vi "read37 and record.vi"(3 "Interval_ms":dbl, 4 "VISA资源名称":refnum<visa-resource-name>) -> (1 "本次记录到的字符串":string)   [LabVIEW 2017]
uses:
  <vilib>/Instr/_visa.llb/VISA Configure Serial Port (Instr).vi
  <vilib>/addons/Tools/Unicode/UTF8 Tools.lvlib
panel:
  out "sensor1":dbl[](array[numeric])
  out "SENSOR21":dbl[](array[numeric])
  out "SENSOR25":dbl[](array[numeric])
  out "SENDSOR13":dbl[](array[numeric])
  out "SENSOR15":dbl[](array[numeric])
  out "SENSOR5":dbl[](array[numeric])
  out "SNESOR3":dbl[](array[numeric])
  out "SENSOR23":dbl[](array[numeric])
  out "SENSOR11":dbl[](array[numeric])
  out "错误输出 2":errorcluster caption="错误输出"
  in  "?":enum32{"CONTROL", "选项卡 2"}(tab)
  in  "增益选择":u16(ring) items=["±6.144V", "±4.096V", "±2.048V", "±1.024V", "±0.512V", "±0.256V"]
  in  "连接方式":u16(ring) items=["Serial", "WiFi", "Dual"]
  out "数值显示控件 37":dbl
  out "数值显示控件":dbl
  out "数值显示控件 2":dbl
  out "数值显示控件 3":dbl
  out "SENSOR11":dbl format="%#.2f"
  out "数值显示控件 5":dbl
  out "数值显示控件 6":dbl
  out "SENSOR13":dbl format="%#.2f"
  out "数值显示控件 8":dbl
  out "数值显示控件 9":dbl
  out "数值显示控件 10":dbl
  out "SENSOR25":dbl format="%#.2f"
  out "数值显示控件 12":dbl
  out "数值显示控件 13":dbl
  out "数值显示控件 14":dbl
  out "SENSOR15":dbl format="%#.2f"
  out "SENSOR5":dbl format="%#.2f"
  out "数值显示控件 17":dbl
  out "数值显示控件 18":dbl
  out "SENSOR23":dbl format="%#.2f"
  out "数值显示控件 20":dbl
  out "数值显示控件 21":dbl
  out "数值显示控件 22":dbl
  out "SENSOR21":dbl format="%#.2f"
  out "数值显示控件 24":dbl
  out "SENSOR1":dbl format="%#.2g"
  out "数值显示控件 26":dbl
  out "数值显示控件 27":dbl
  out "数值显示控件 28":dbl
  out "数值显示控件 29":dbl
  out "数值显示控件 30":dbl
  out "SENSOR3":dbl format="%#.2f"
  out "数值显示控件 32":dbl
  out "数值显示控件 33":dbl
  out "数值显示控件 34":dbl
  out "数值显示控件 35":dbl
  out "数值显示控件 36":dbl
  out "本次":string
  out "finally":string[][](array[string])
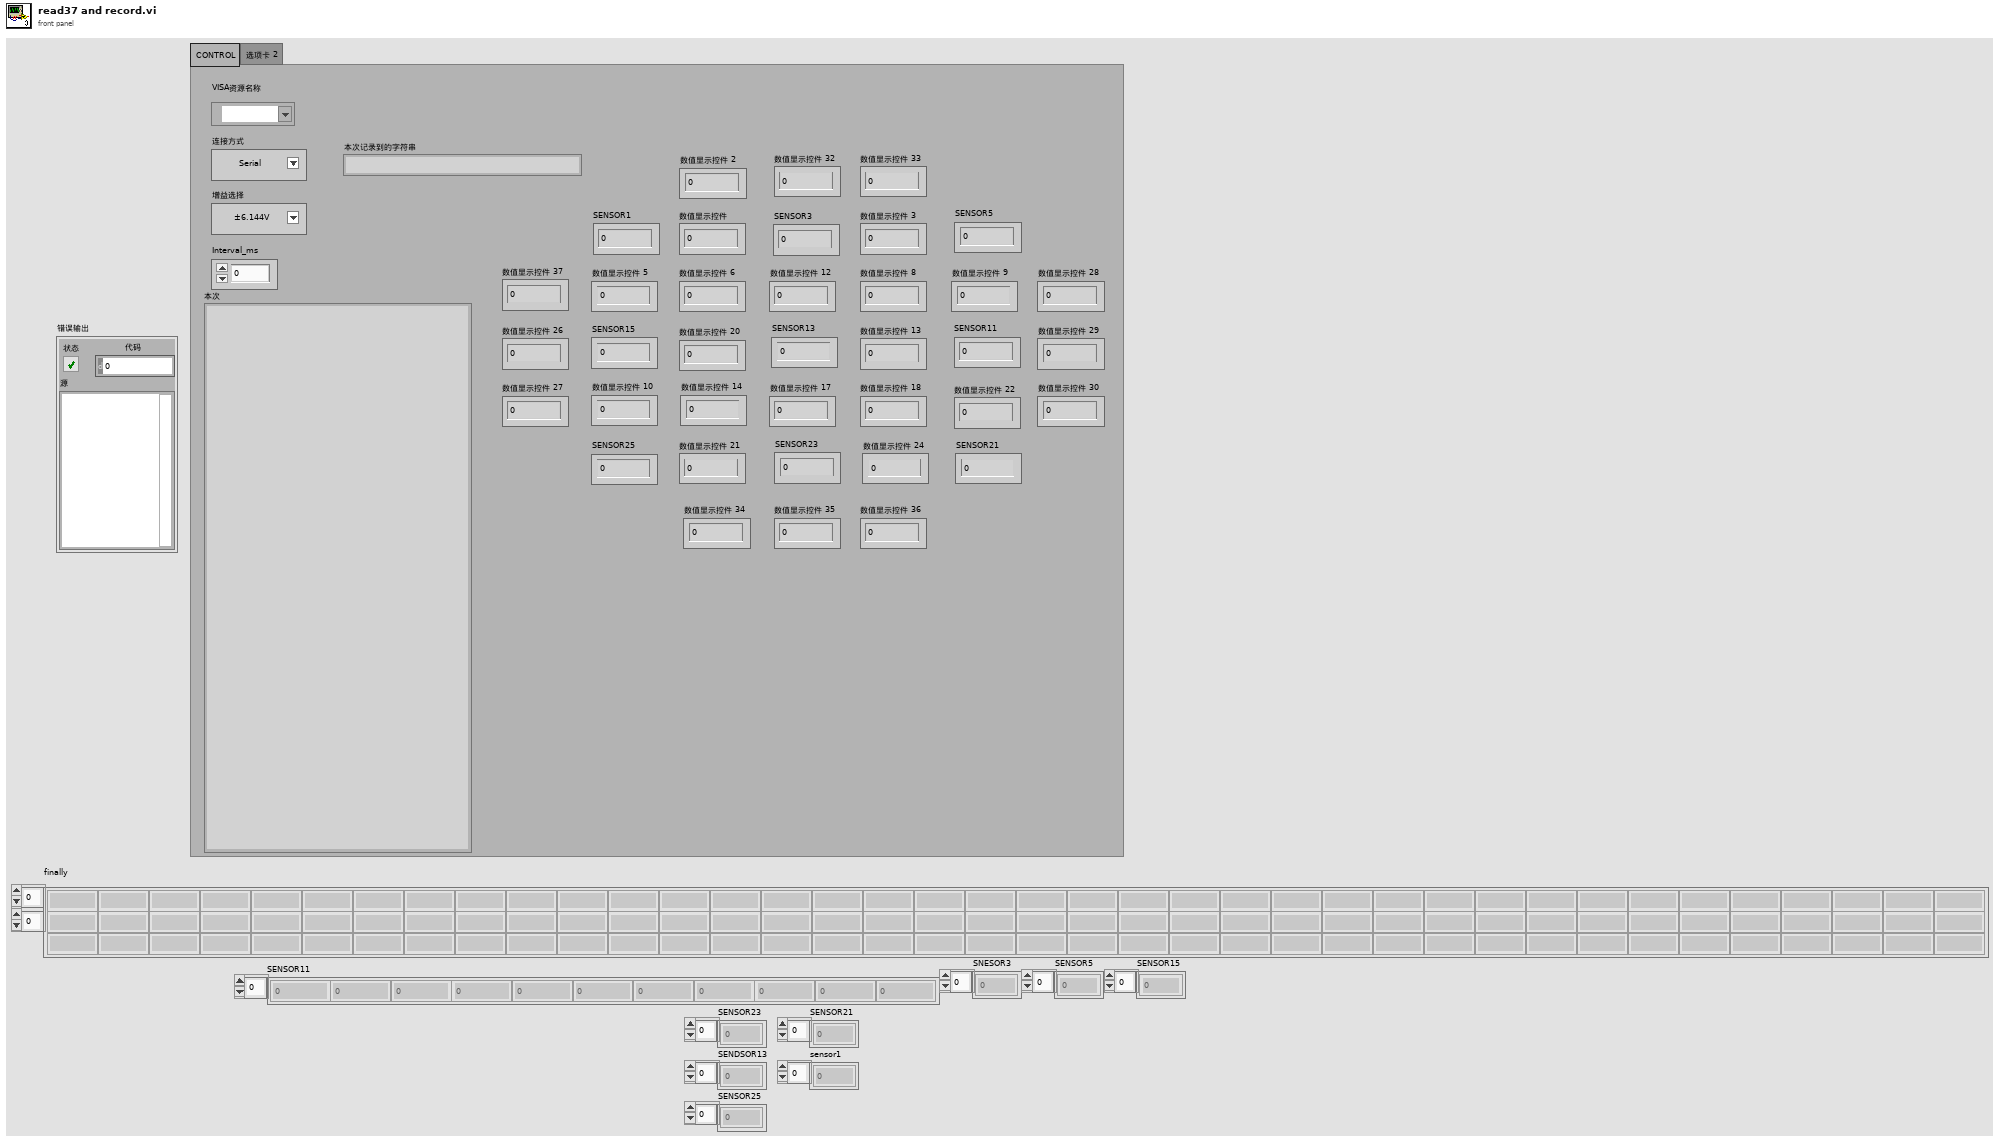
[diagram p1: front panel]
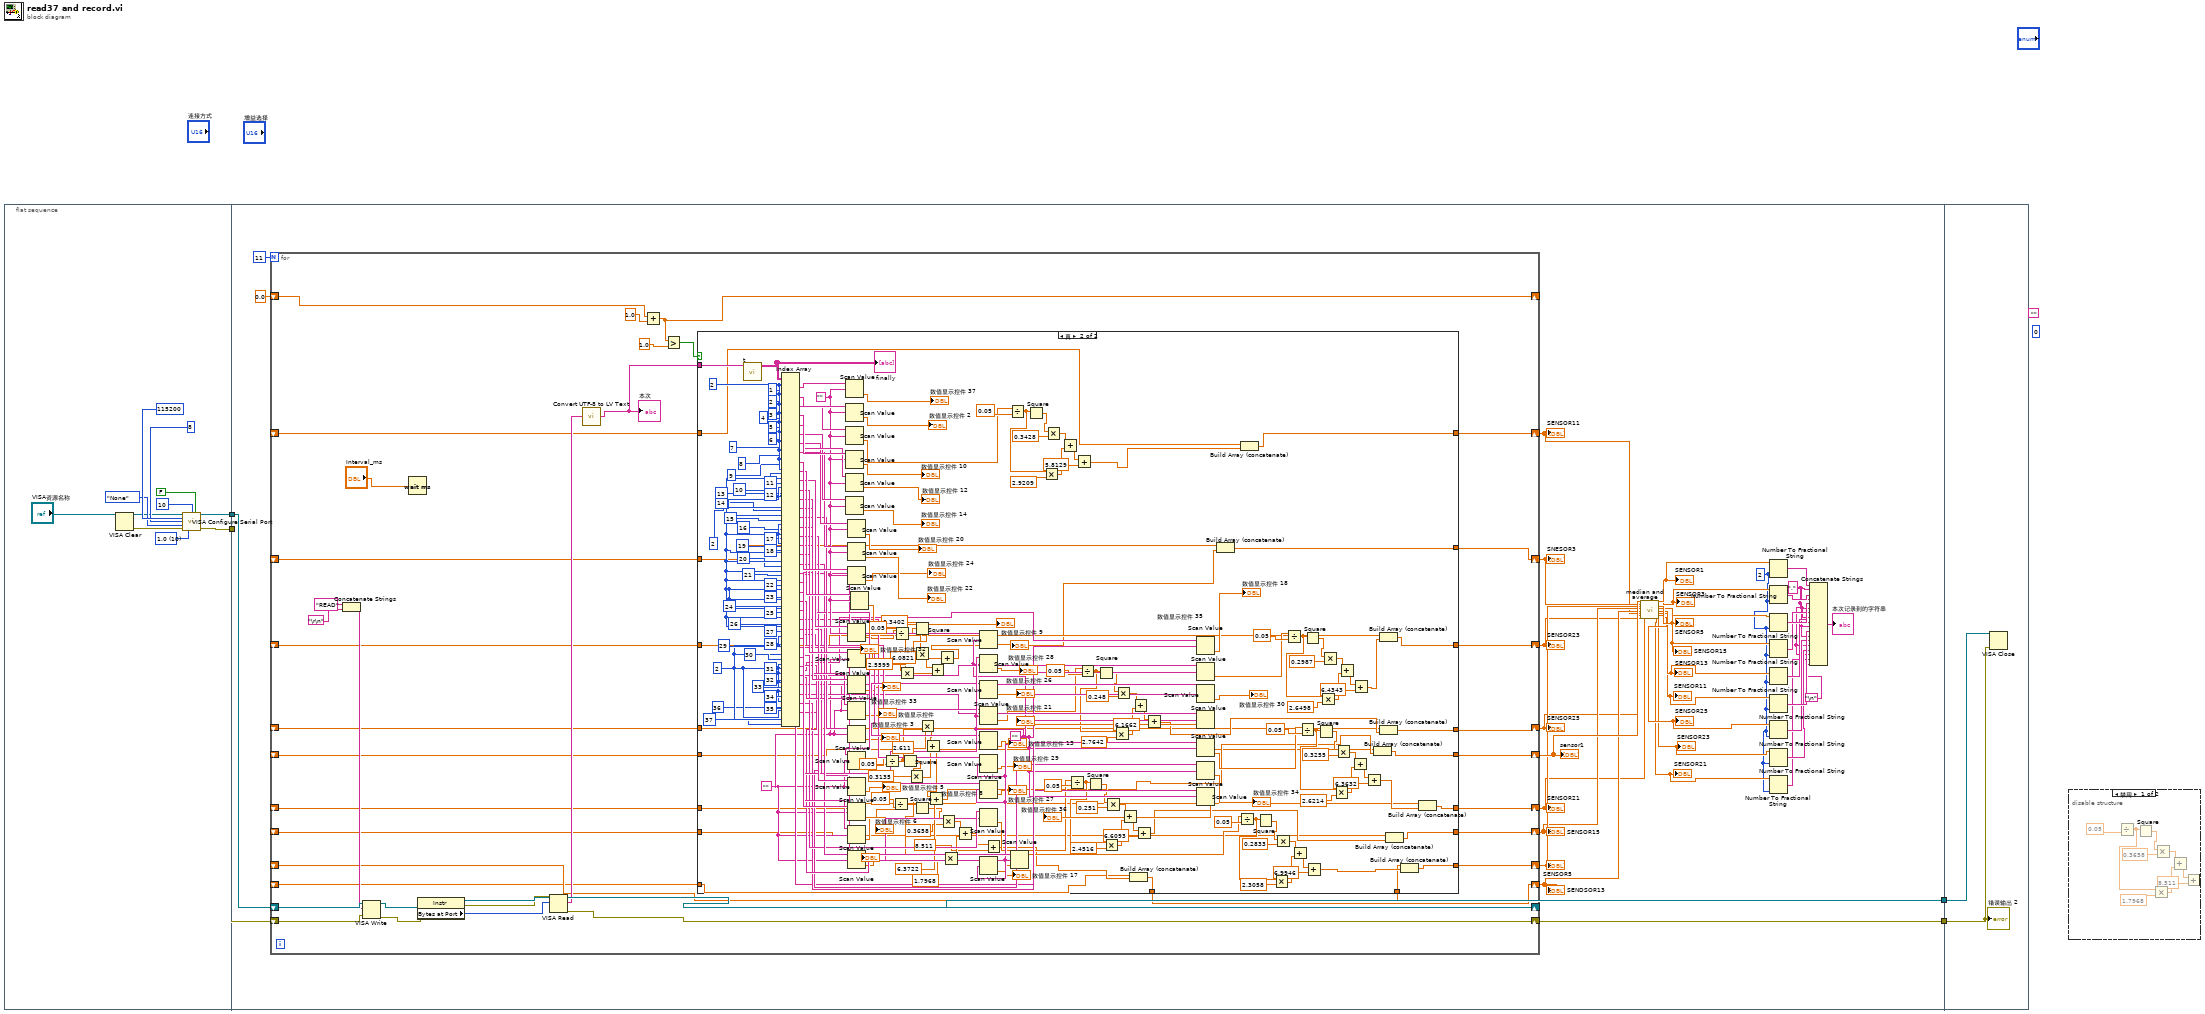
[diagram p0: block diagram]
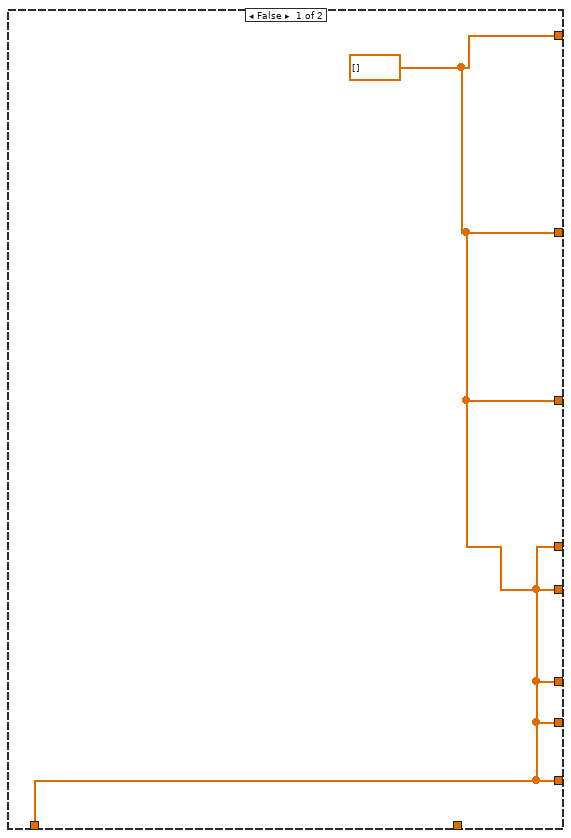
[diagram p3: hidden frame]
diagram:
  (unwired) 0
  (unwired) ""
  n1 = flat-sequence {
    tunnel: [w7] -> w4
    tunnel: [w6] -> w3
    tunnel: w4 -> [w52]
    tunnel: w3 -> [w51]
    tunnel: [w50] -> w2
    tunnel: [w49] -> w1
    tunnel: w2 -> [w320]
    tunnel: w1 -> [w319]
    frame #0 {
      w14 = u16 10 items=["1.0"=10, "1.5"=15, "2.0"=20] ("stop bits (10: 1 bit)")
      n2 = VISA Clear(VISA resource name="VISA资源名称") -> (VISA resource name out=w10:refnum<visa-resource-name>, error out=w9:errorcluster)  [unwired: 1 in]
      n3 = call-poly "VISA Configure Serial Port"("VISA resource name"=w10, "termination char\n(0xA = '\\n' = LF)"=u8 10 ("termination char\n(0xA = '\\n' = LF)"), "Enable Termination\nChar (T)"=FALSE ("Enable Termination\nChar (T)"), "baud rate (9600)"=u32 115200, "data bits (8)"=u16 8, "parity (0:none)"=enum16{"None", "Odd", "Even", "Mark", "Space"}."None", "error in (no error)"=w9, "stop bits (10: 1 bit)"=w14) -> ("VISA resource name out"=w6:refnum<visa-resource-name>, "error out"=w7:errorcluster)  [unwired: 6 in]
    }
    frame #1 {
      w16 = i16 2 ("精度(6)")
      w19 = "," ("字符串")
      n4 = for {
        N: 11 -> [_]
        shift-right: [w87] -> w49
        shift-left: w52 -> [w90]
        shift-right: [w88] -> w50
        shift-left: w51 -> [w89]
        shift-right: [w77] -> _
        shift-left: 0.0 -> [w78]
        shift-right: [w70] -> w41
        shift-left: _ -> [w69]
        shift-right: [w68] -> w39
        shift-left: _ -> [w67]
        shift-right: [w66] -> w45
        shift-left: _ -> [w65]
        shift-right: [w64] -> w44
        shift-left: _ -> [w63]
        shift-right: [w62] -> w43
        shift-left: _ -> [w61]
        shift-right: [w60] -> w42
        shift-left: _ -> [w59]
        shift-right: [w58] -> w40
        shift-left: _ -> [w57]
        shift-right: [w56] -> w38
        shift-left: _ -> [w55]
        shift-right: [w54] -> w46
        shift-left: _ -> [w53]
        n5 = Concatenate Strings("READ" ("字符串"), "\r\n") -> (w86:string)
        n6 = VISA Write(VISA resource name=w89, write buffer=w86, error in (no error)=w90) -> (VISA resource name out=w85:refnum<visa-resource-name>, error out=w84:errorcluster)  [unwired: 1 out]
        n7 = Wait (ms)(milliseconds to wait="Interval_ms") -> ()  [unwired: 1 out]
        n8 = property class="Instr"(reference=w85, error in=w84) -> (reference out=w82:refnum<visa-resource-name>, error out=w81:errorcluster, "Bytes at Port"=w80:u32)
        n9 = VISA Read(VISA resource name=w82, byte count=w80, error in (no error)=w81) -> (VISA resource name out=w88:refnum<visa-resource-name>, read buffer=w79:string, error out=w87:errorcluster)  [unwired: 1 out]
        n10 = call <vilib>:"Convert UTF-8 to LV Text.vi"("UTF-8 Text"=w79) -> ("LV Text"=w71:string)  [unwired: 13 in, 1 out]
        "本次" <- w71
        n11 = Add(x=w78, y=1.0) -> (x+y=w77:dbl)
        n12 = Greater?(x=w77, y=1.0) -> (0:w74:bool)
        n13 = case shown="真" w74 {
          tunnel: w71 -> [_ w119]
          tunnel: [w91 w118] -> w70
          tunnel: w69 -> [_ w117]
          tunnel: [w91 w116] -> w68
          tunnel: w67 -> [_ w114]
          tunnel: [w91 w113] -> w66
          tunnel: w65 -> [_ w111]
          tunnel: [w91 w110] -> w64
          tunnel: w63 -> [_ w108]
          tunnel: [w91 w107] -> w62
          tunnel: w61 -> [_ w105]
          tunnel: [w91 w104] -> w60
          tunnel: w59 -> [_ w102]
          tunnel: [w91 w101] -> w58
          tunnel: w57 -> [_ w99]
          tunnel: [w91 w97] -> w56
          tunnel: w55 -> [_ w96]
          tunnel: [w91 w95] -> w54
          tunnel: w53 -> [_ w93]
          frame False {
            w91 = dbl[] []
          }
          frame True {
            w229 = ""
            w230 = ""
            w261 = 2 ("索引 (行)")
            w287 = 2 ("索引 (行)")
            w257 = ""
            w317 = 2 ("索引 (行)")
            n14 = call "t.vi"("待处理字符串"=w119) -> ("finally"=w318:string[][])  [unwired: 10 in]
            "finally" <- w318
            n15 = Index Array(array=w318, index (row) #1=w317, index (col) #1=1 ("禁用的索引 (列)"), index (row) #2=w317, index (col) #2=2 ("禁用的索引 (列)"), index (row) #3=w317, index (col) #3=3 ("禁用的索引 (列)"), index (row) #4=w317, index (col) #4=4 ("禁用的索引 (列)"), index (row) #5=w317, index (col) #5=5 ("禁用的索引 (列)"), index (row) #6=w317, index (col) #6=6 ("禁用的索引 (列)"), index (row) #7=w317, index (col) #7=7 ("禁用的索引 (列)"), index (row) #8=w317, index (col) #8=8 ("禁用的索引 (列)"), index (row) #9=w317, index (col) #9=9 ("禁用的索引 (列)"), index (row) #10=w317, index (col) #10=10 ("禁用的索引 (列)"), index (row) #11=w287, index (col) #11=11 ("禁用的索引 (列)"), index (row) #12=w287, index (col) #12=12 ("禁用的索引 (列)"), index (row) #13=w287, index (col) #13=13 ("禁用的索引 (列)"), index (row) #14=w287, index (col) #14=14 ("禁用的索引 (列)"), index (row) #15=w287, index (col) #15=15 ("禁用的索引 (列)"), index (row) #16=w287, index (col) #16=16 ("禁用的索引 (列)"), index (row) #17=w287, index (col) #17=17 ("禁用的索引 (列)"), index (row) #18=w287, index (col) #18=18 ("禁用的索引 (列)"), index (row) #19=w287, index (col) #19=19 ("禁用的索引 (列)"), index (row) #20=w287, index (col) #20=20 ("禁用的索引 (列)"), index (row) #21=w287, index (col) #21=21 ("禁用的索引 (列)"), index (row) #22=w287, index (col) #22=22 ("禁用的索引 (列)"), index (row) #23=w287, index (col) #23=23 ("禁用的索引 (列)"), index (row) #24=w287, index (col) #24=24 ("禁用的索引 (列)"), index (row) #25=w287, index (col) #25=25 ("禁用的索引 (列)"), index (row) #26=w287, index (col) #26=26 ("禁用的索引 (列)"), index (row) #27=w287, index (col) #27=27 ("禁用的索引 (列)"), index (row) #28=w261, index (col) #28=28 ("禁用的索引 (列)"), index (row) #29=w261, index (col) #29=29 ("禁用的索引 (列)"), index (row) #30=w261, index (col) #30=30 ("禁用的索引 (列)"), index (row) #31=w261, index (col) #31=31 ("禁用的索引 (列)"), index (row) #32=w261, index (col) #32=32 ("禁用的索引 (列)"), index (row) #33=w261, index (col) #33=33 ("禁用的索引 (列)"), index (row) #34=w261, index (col) #34=34 ("禁用的索引 (列)"), index (row) #35=w261, index (col) #35=35 ("禁用的索引 (列)"), index (row) #36=w261, index (col) #36=36 ("禁用的索引 (列)"), index (row) #37=w261, index (col) #37=37 ("禁用的索引 (列)")) -> (element #1=w309:string, element #2=w308:string, element #3=w307:string, element #4=w306:string, element #5=w305:string, element #6=w304:string, element #7=w303:string, element #8=w302:string, element #9=w298:string, element #10=w297:string, element #11=w258:string, element #12=w256:string, element #13=w255:string, element #14=w254:string, element #15=w253:string, element #16=w252:string, element #17=w251:string, element #18=w250:string, element #19=w249:string, element #20=w248:string, element #21=w247:string, element #22=w246:string, element #23=w245:string, element #24=w244:string, element #25=w243:string, element #26=w242:string, element #27=w241:string, element #28=w240:string, element #29=w239:string, element #30=w238:string, element #31=w237:string, element #32=w236:string, element #33=w235:string, element #34=w234:string, element #35=w233:string, element #36=w232:string, element #37=w231:string)
            n16 = Scan Value(string=w309, format string=w257) -> (value=→"数值显示控件 37":dbl)  [unwired: 1 in, 1 out]
            n17 = Scan Value(string=w308, format string=w257) -> (value=→"数值显示控件 2":dbl)  [unwired: 1 in, 1 out]
            n18 = Scan Value(string=w307, format string=w257) -> (value=w151:dbl)  [unwired: 1 in, 1 out]
            n19 = Scan Value(string=w306, format string=w257) -> (value=→"数值显示控件 10":dbl)  [unwired: 1 in, 1 out]
            n20 = Scan Value(string=w305, format string=w257) -> (value=→"数值显示控件 12":dbl)  [unwired: 1 in, 1 out]
            n21 = Scan Value(string=w304, format string=w257) -> (value=→"数值显示控件 14":dbl)  [unwired: 1 in, 1 out]
            n22 = Scan Value(string=w303, format string=w257) -> (value=→"数值显示控件 20":dbl)  [unwired: 1 in, 1 out]
            n23 = Scan Value(string=w302, format string=w257) -> (value=→"数值显示控件 22":dbl)  [unwired: 1 in, 1 out]
            n24 = Scan Value(string=w298, format string=w257) -> (value=→"数值显示控件 24":dbl)  [unwired: 1 in, 1 out]
            n25 = Scan Value(string=w258, format string=w257) -> (value=w199:dbl)  [unwired: 1 in, 1 out]
            n26 = Scan Value(string=w256, format string=w230) -> (value=→"数值显示控件 32":dbl)  [unwired: 1 in, 1 out]
            n27 = Scan Value(string=w255, format string=w230) -> (value=→"数值显示控件 33":dbl)  [unwired: 1 in, 1 out]
            n28 = Scan Value(string=w254, format string=w230) -> (value=→"数值显示控件":dbl)  [unwired: 1 in, 1 out]
            n29 = Scan Value(string=w253, format string=w230) -> (value=→"数值显示控件 3":dbl)  [unwired: 1 in, 1 out]
            n30 = Scan Value(string=w252, format string=w230) -> (value=w209:dbl)  [unwired: 1 in, 1 out]
            n31 = Scan Value(string=w251, format string=w230) -> (value=→"数值显示控件 5":dbl)  [unwired: 1 in, 1 out]
            n32 = Scan Value(string=w250, format string=w230) -> (value=→"数值显示控件 6":dbl)  [unwired: 1 in, 1 out]
            n33 = Scan Value(string=w249, format string=w230) -> (value=w161:dbl)  [unwired: 1 in, 1 out]
            n34 = Scan Value(string=w248, format string=w230) -> (value=→"数值显示控件 8":dbl)  [unwired: 1 in, 1 out]
            n35 = Scan Value(string=w297, format string=w257) -> (value=→"数值显示控件 35":dbl)  [unwired: 1 in, 1 out]
            n36 = Divide(x=w209, y=0.05) -> (x/y=w204:dbl)
            n37 = Divide(x=w161, y=0.05) -> (x/y=w168:dbl)
            n38 = Divide(x=w199, y=0.05) -> (x/y=w194:dbl)
            n39 = Multiply(x=w194, y=2.5599) -> (x*y=w192:dbl)
            n40 = Square(x=w204) -> (x^2=w207:dbl)
            n41 = Multiply(x=w207, y=0.3135) -> (x*y=w205:dbl)
            n42 = Square(x=w194) -> (x^2=w197:dbl)
            n43 = Multiply(x=w197, y=0.3402) -> (x*y=w195:dbl)
            n44 = Square(x=w168) -> (x^2=w166:dbl)
            n45 = Multiply(x=2.611, y=w204) -> (x*y=w202:dbl)
            n46 = Add(x=w202, y=w205) -> (x+y=w201:dbl)
            n47 = Add(x=w201, y=6.3722) -> (x+y=w94:dbl)
            n48 = Add(x=w195, y=w192) -> (x+y=w191:dbl)
            n49 = Add(x=6.0821, y=w191) -> (x+y=w112:dbl)
            n50 = Multiply(x=w166, y=0.3658) -> (x*y=w167:dbl)
            n51 = Multiply(x=w168, y=1.7968) -> (x*y=w169:dbl)
            n52 = Add(x=w167, y=w169) -> (x+y=w120:dbl)
            n53 = Scan Value(string=w247, format string=w229) -> (value=→"数值显示控件 9":dbl)  [unwired: 1 in, 1 out]
            n54 = Scan Value(string=w246, format string=w229) -> (value=→"数值显示控件 28":dbl)  [unwired: 1 in, 1 out]
            n55 = Scan Value(string=w245, format string=w229) -> (value=→"数值显示控件 26":dbl)  [unwired: 1 in, 1 out]
            n56 = Scan Value(string=w244, format string=w229) -> (value=w141:dbl)  [unwired: 1 in, 1 out]
            n57 = Scan Value(string=w243, format string=w229) -> (value=→"数值显示控件 13":dbl)  [unwired: 1 in, 1 out]
            n58 = Scan Value(string=w242, format string=w229) -> (value=→"数值显示控件 29":dbl)  [unwired: 1 in, 1 out]
            n59 = Scan Value(string=w241, format string=w229) -> (value=→"数值显示控件 27":dbl)  [unwired: 1 in, 1 out]
            n60 = Scan Value(string=w240, format string=w229) -> (value=w170:dbl)  [unwired: 1 in, 1 out]
            n61 = Scan Value(string=w238, format string=w229) -> (value=→"数值显示控件 17":dbl)  [unwired: 1 in, 1 out]
            n62 = Add(x=w120, y=8.511) -> (x+y=w103:dbl)
            n63 = Divide(x=w151, y=0.05) -> (x/y=w156:dbl)
            n64 = Scan Value(string=w239, format string=w229) -> (value=w180:dbl)  [unwired: 1 in, 1 out]
            n65 = Square(x=w156) -> (x^2=w159:dbl)
            n66 = Multiply(x=w156, y=2.9209) -> (x*y=w154:dbl)
            n67 = Multiply(x=w159, y=0.3428) -> (x*y=w157:dbl)
            n68 = Add(x=w157, y=w154) -> (x+y=w153:dbl)
            n69 = Divide(x=w170, y=0.05) -> (x/y=w175:dbl)
            n70 = Add(x=w153, y=5.8129) -> (x+y=w92:dbl)
            n71 = Divide(x=w141, y=0.05) -> (x/y=w147:dbl)
            n72 = Square(x=w175) -> (x^2=w178:dbl)
            n73 = Square(x=w147) -> (x^2=w150:dbl)
            n74 = Multiply(x=w175, y=2.4516) -> (x*y=w173:dbl)
            n75 = Multiply(x=w178, y=0.251) -> (x*y=w176:dbl)
            n76 = Multiply(x=w147, y=2.7642) -> (x*y=w145:dbl)
            n77 = Multiply(x=w150, y=0.248) -> (x*y=w148:dbl)
            n78 = Add(x=w176, y=w173) -> (x+y=w172:dbl)
            n79 = Build Array (concatenate)(w102, w103) -> (w104:dbl[])
            n80 = Add(x=w148, y=w145) -> (x+y=w144:dbl)
            n81 = Add(x=w172, y=6.6093) -> (x+y=w106:dbl)
            n82 = Add(x=w144, y=6.1662) -> (x+y=w100:dbl)
            n83 = Scan Value(string=w237, format string=w229) -> (value=→"数值显示控件 18":dbl)  [unwired: 1 in, 1 out]
            n84 = Scan Value(string=w236, format string=w229) -> (value=w131:dbl)  [unwired: 1 in, 1 out]
            n85 = Scan Value(string=w235, format string=w229) -> (value=→"数值显示控件 30":dbl)  [unwired: 1 in, 1 out]
            n86 = Scan Value(string=w234, format string=w229) -> (value=→"数值显示控件 21":dbl)  [unwired: 1 in, 1 out]
            n87 = Scan Value(string=w233, format string=w229) -> (value=w121:dbl)  [unwired: 1 in, 1 out]
            n88 = Scan Value(string=w232, format string=w229) -> (value=→"数值显示控件 34":dbl)  [unwired: 1 in, 1 out]
            n89 = Scan Value(string=w231, format string=w229) -> (value=→"数值显示控件 36":dbl)  [unwired: 1 in, 1 out]
            n90 = Build Array (concatenate)(w111, w112) -> (w113:dbl[])
            n91 = Divide(x=w180, y=0.05) -> (x/y=w185:dbl)
            n92 = Build Array (concatenate)(w117, w92) -> (w118:dbl[])
            n93 = Square(x=w185) -> (x^2=w188:dbl)
            n94 = Multiply(x=w185, y=2.3058) -> (x*y=w183:dbl)
            n95 = Multiply(x=w188, y=0.2833) -> (x*y=w186:dbl)
            n96 = Divide(x=w131, y=0.05) -> (x/y=w138:dbl)
            n97 = Add(x=w186, y=w183) -> (x+y=w182:dbl)
            n98 = Divide(x=w121, y=0.05) -> (x/y=w128:dbl)
            n99 = Square(x=w138) -> (x^2=w136:dbl)
            n100 = Add(x=w182, y=6.9946) -> (x+y=w109:dbl)
            n101 = Square(x=w128) -> (x^2=w126:dbl)
            n102 = Multiply(x=w138, y=2.6498) -> (x*y=w139:dbl)
            n103 = Multiply(x=w136, y=0.2987) -> (x*y=w137:dbl)
            n104 = Multiply(x=w128, y=2.6214) -> (x*y=w129:dbl)
            n105 = Multiply(x=w126, y=0.3255) -> (x*y=w127:dbl)
            n106 = Add(x=w137, y=w139) -> (x+y=w140:dbl)
            n107 = Add(x=w127, y=w129) -> (x+y=w130:dbl)
            n108 = Add(x=w140, y=6.4343) -> (x+y=w115:dbl)
            n109 = Add(x=w130, y=6.3632) -> (x+y=w98:dbl)
            n110 = Build Array (concatenate)(w93, w94) -> (w95:dbl[])
            n111 = Build Array (concatenate)(w114, w115) -> (w116:dbl[])
            n112 = Build Array (concatenate)(w99, w100) -> (w101:dbl[])
            n113 = Build Array (concatenate)(w105, w106) -> (w107:dbl[])
            n114 = Build Array (concatenate)(w108, w109) -> (w110:dbl[])
            n115 = Build Array (concatenate)(w96, w98) -> (w97:dbl[])
          }
        }
      }
      "SENSOR11" <- w41
      "SENSOR23" <- w39
      "SNESOR3" <- w45
      "SENSOR5" <- w44
      "SENSOR15" <- w43
      "SENDSOR13" <- w42
      "SENSOR25" <- w40
      "SENSOR21" <- w38
      "sensor1" <- w46
      n116 = call "median and average.vi"("sensor 1"=w46, "sensor2"=w45, "sensor3"=w44, "sensor 4"=w43, "sensor 5"=w42, "sensor 6"=w41, "sensor 7"=w40, "sensor 8"=w39, "sensor 9"=w38) -> ("9"=w28:dbl, "1"=w36:dbl, "2"=w35:dbl, "3"=w34:dbl, "4"=w33:dbl, "5"=w32:dbl, "6"=w31:dbl, "7"=w30:dbl, "8"=w29:dbl)  [unwired: 10 in]
      "SENSOR1" <- w36
      "SENSOR3" <- w35
      "SENSOR5" <- w34
      "SENSOR15" <- w33
      "SENSOR13" <- w32
      "SENSOR11" <- w31
      "SENSOR25" <- w30
      "SENSOR23" <- w29
      "SENSOR21" <- w28
      n117 = Number To Fractional String(number=w36, precision (6)=w16) -> (F-format string=w37:string)  [unwired: 2 in]
      n118 = Number To Fractional String(number=w35, precision (6)=w16) -> (F-format string=w27:string)  [unwired: 2 in]
      n119 = Number To Fractional String(number=w34, precision (6)=w16) -> (F-format string=w26:string)  [unwired: 2 in]
      n120 = Number To Fractional String(number=w33, precision (6)=w16) -> (F-format string=w25:string)  [unwired: 2 in]
      n121 = Number To Fractional String(number=w32, precision (6)=w16) -> (F-format string=w24:string)  [unwired: 2 in]
      n122 = Number To Fractional String(number=w31, precision (6)=w16) -> (F-format string=w23:string)  [unwired: 2 in]
      n123 = Number To Fractional String(number=w30, precision (6)=w16) -> (F-format string=w22:string)  [unwired: 2 in]
      n124 = Number To Fractional String(number=w29, precision (6)=w16) -> (F-format string=w21:string)  [unwired: 2 in]
      n125 = Number To Fractional String(number=w28, precision (6)=w16) -> (F-format string=w20:string)  [unwired: 2 in]
      n126 = Concatenate Strings(w37, w19, w27, w19, w26, w19, w25, w19, w24, w19, w23, w19, w22, w19, w21, w19, w20, "\n") -> (→"本次记录到的字符串":string)
    }
    frame #2 {
      n127 = VISA Close(VISA resource name=w320, error in (no error)=w319) -> ()  [unwired: 1 out]
      "错误输出 2" <- w319
    }
  }
  n128 = disable-structure shown="禁用" {
    frame Disabled {
      n129 = Divide(y=0.05) -> (x/y=w325:dbl)  [unwired: 1 in]
      n130 = Square(x=w325) -> (x^2=w328:dbl)
      n131 = Multiply(x=w325, y=1.7968) -> (x*y=w323:dbl)
      n132 = Multiply(x=w328, y=0.3658) -> (x*y=w326:dbl)
      n133 = Add(x=w326, y=w323) -> (x+y=w322:dbl)
      n134 = Add(x=w322, y=8.511) -> ()  [unwired: 1 out]
    }
    frame Enabled {
    }
  }
